vi "RollingGradient.vi"(8 "TempArray in":dbl[](array[numeric]), 9 "FitSize":i32, 10 "dt":dbl, 11 "mean temp":dbl) -> (0 "TempArray":dbl[](array[numeric]), 3 "gradient":dbl)   [LabVIEW 2021]
uses:
  <vilib>/Analysis/NI_AALPro.lvlib
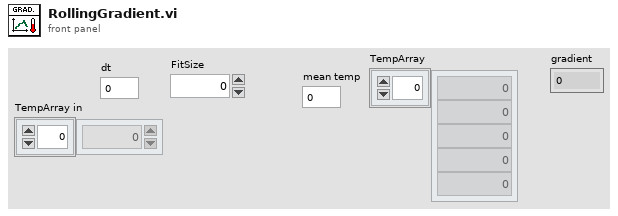
[diagram p1: front panel]
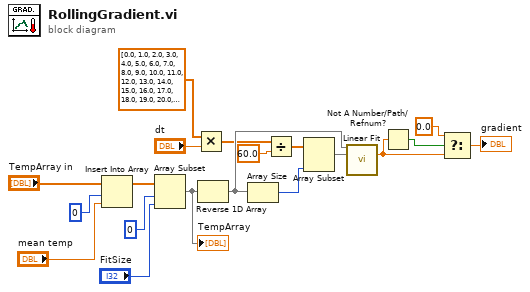
[diagram p0: block diagram]
diagram:
  n1 = Insert Into Array(array="TempArray in", index=0, new element="mean temp") -> (w18:dbl[])
  n2 = Array Subset(array=w18, index=0, length="FitSize") -> (w15:dbl[])
  "TempArray" <- w15
  n3 = Multiply(x=dbl[] [0.0, 1.0, 2.0, 3.0, 4.0, 5.0, 6.0, 7.0, 8.0, 9.0, 10.0, 11.0, 12.0, 13.0, 14.0, 15.0, 16.0, 17.0, 18.0, 19.0, 20.0, 21.0, 22.0, 23.0, 24.0, 25.0, 26.0, 27.0, 28.0, 29.0, 30.0], y="dt") -> (x*y=w13:dbl[])
  n4 = Reverse 1D Array(array=w15) -> (reversed array=w14:dbl[])
  n5 = Array Size(array=w14) -> (size(s)=w11:i32)
  n6 = Divide(x=w13, y=60.0) -> (x/y=w7:dbl[])
  n7 = Array Subset(array=w7, length=w11) -> (w12:dbl[])  [unwired: 1 in]
  n8 = call <vilib>:"Linear Fit.vi"("Y"=w14, "X"=w12) -> ("slope"=w3:dbl)  [unwired: 9 in, 4 out]
  n9 = Not A Number/Path/Refnum?(number/path/refnum=w3) -> (NaN/Path/Refnum?=w4:bool)
  n10 = Select(t=0.0, s=w4, f=w3) -> (s? t:f=→"gradient":dbl)
